vi "Rinocloud_browser.vi"() -> ()   [LabVIEW 2013, in "Rinocloud Library.lvlib"]
uses:
  Rinocloud Library.lvlib
  Rinocloud API endpoint VIs/API_endpoint_subVIs/State_Control.ctl
  Rinocloud_global_variable.vi
panel:
  in  "page indicator":string
  in  "Next page":bool
  in  "Previous page":bool
  out "Last action:":string
  in  "Active item:":string="<folder> home (id=)"
  in  "delete":bool
  in  "refresh list":bool
  in  "Tab Control":T1(tab)=enum."Inspect"
  in  "Cluster 2":T2={"Attribute"="", "Value"="", "Data type"=5} {"Data type" items=["Numeric", "String", "1D array of strings", "1D array of doubles", "Data JSON string", "<null>"]}
  in  "Cluster 1":T2={"Attribute"="", "Value"="", "Data type"=5} {"Data type" items=["Numeric", "String", "1D array of strings", "1D array of doubles", "Data JSON string", "<null>"]}
  in  "name":string
  in  "tags":string
  in  "notes":string
  in  "new folder":bool
  in  "upload file":bool
  in  "Store data locally":bool
  in  "Store metadata locally":bool
  in  "Name:":string
  in  "Tags:":string
  in  "Notes:":string
  in  "get metadata":bool
  in  "metadata tree":string(tree) caption="Metadata"
  in  "update metadata":bool
  in  "Move":bool
  in  "Destination:":string
  in  "Source:":string
  in  "set source":bool
  in  "set destination":bool
  out "body":string
  out "headers":string
  in  "error message":string caption="Error:"
  in  "ancestor tree":string(tree)="home" caption="Active path"
  in  "stop":bool
  in  "active child tree":string(tree) caption="File & folder list of the active folder"
  # "Double-click an item to activate"
  # "Custom metadata:"
  # "(tag1,tag2,tag3,...)"
  # "Click the fields to edit"
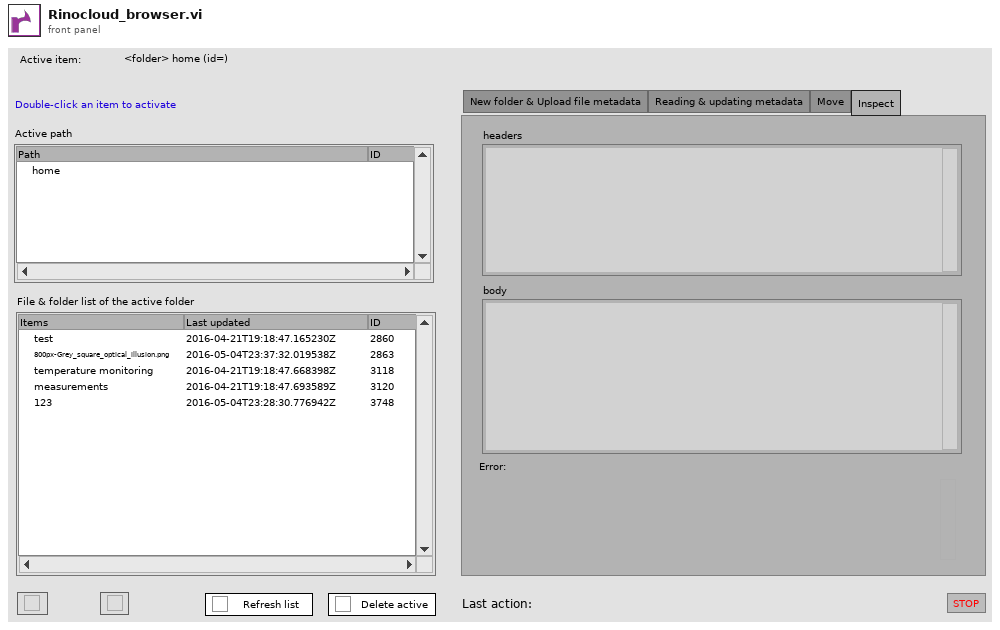
[diagram p1: front panel]
types:
  T1 = enum32{"New folder & Upload file metadata", "Reading & updating metadata", "Move", "Inspect"}
  T2 = cluster{"Attribute":string, "Value":string, "Data type":u16}
  T3 = cluster{"Active items":cluster{"Active file ID":string, "Active dir ID":string, "Active object ID":string, "Recent ID":string, "Active item:":string, "Source item":string, "Destination item":string, "Source ID":string, "Destination ID":string}, "Trees":cluster{"Ancestors":refnum<vi>, "Children":refnum<vi>, "Metadata":refnum<vi>}, "New metadata":cluster{"Name":string, "Tags":string, "Notes":string, "Custom metadata":cluster{"Attribute":string, "Value":string, "Data type":u16}[]}, "Communication":cluster{"HTTP headers":string, "HTTP body":string, "Project name":string, "User":string, "HTTP ch body":string}, "Controls":cluster{"Move refnum":refnum<vi>}, "Status messages":cluster{"error ":errorcluster, "status":string}, "Update metadata":cluster{"Name":string, "Tags":string, "Notes":string}, "Pagination":cluster{"total":dbl, "limit":dbl, "offset":dbl, "count":dbl, " next page refnum":refnum<vi>, "previous page refnum":refnum<vi>, "page indicator":string}}
  T4 = typedef "State_Control.ctl" = enum16{"Boot", "Initialize", "Wait for event", "Refresh", "Pagination", "Metadata to tree", "Stop"}
  T5 = cluster{"HTTP headers":string, "HTTP body":string, "Project name":string, "User":string, "HTTP ch body":string}
  T6 = cluster{"Active file ID":string, "Active dir ID":string, "Active object ID":string, "Recent ID":string, "Active item:":string, "Source item":string, "Destination item":string, "Source ID":string, "Destination ID":string}
  T7 = enum8{"Enabled", "Disabled", "Disabled and Grayed Out"}
  T8 = cluster{"Name":string, "Tags":string, "Notes":string, "Custom metadata":cluster{"Attribute":string, "Value":string, "Data type":u16}[]}
  T9 = enum16{"Boot", "Initialize", "Wait for event", "Refresh", "Pagination", "Metadata to tree", "Stop"}
  T10 = cluster{"Store locally":bool, "ancestor array":cluster{"id":string, "name":string, "created_on":string, "updated_on":string, "tags":string, "notes":string, "record type":string, "metadata (JSON)":string}[], "Store metadata":bool}
  T11 = cluster{"Attribute":string, "Value":string, "Data type":enum16{"Numeric", "String", "1D array of strings", "1D array of doubles", "Data JSON string", "<null>"}}[]
  T12 = cluster{"limit":dbl, "total":dbl, "offset":dbl, "count":dbl}
  T13 = cluster{"headers":string, "body":string, "ID":string, "Saved":bool}
  T14 = cluster{"Attribute":string, "Value":string, "Data type":u16}[]
  T15 = cluster{"id":string, "name":string, "created_on":string, "updated_on":string, "tags":string, "notes":string, "record type":string, "metadata (JSON)":string}[]
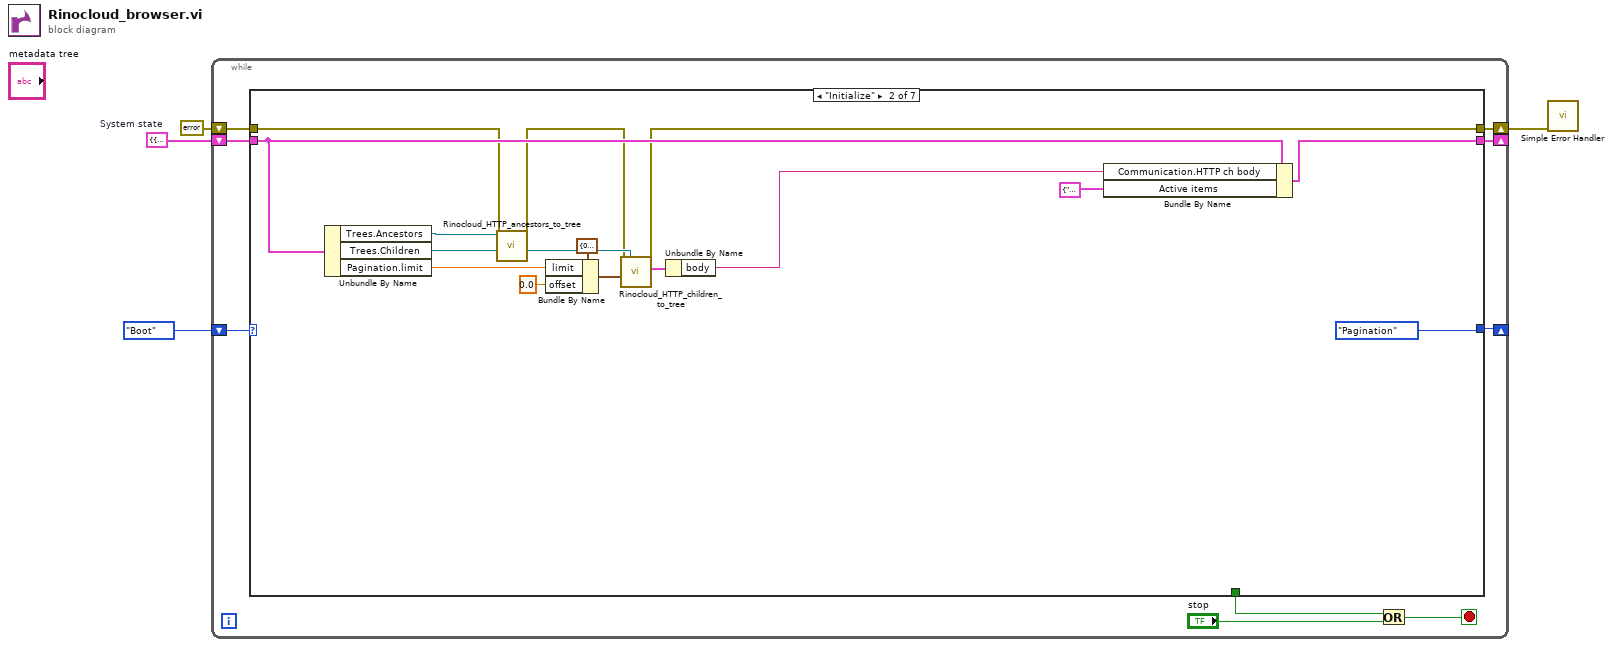
[diagram p0: block diagram]
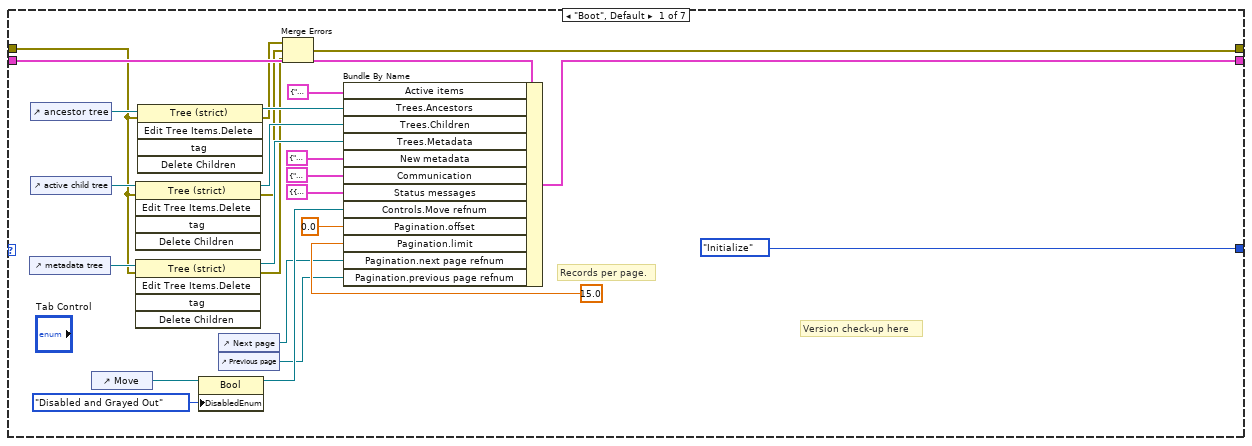
[diagram p2: hidden frame]
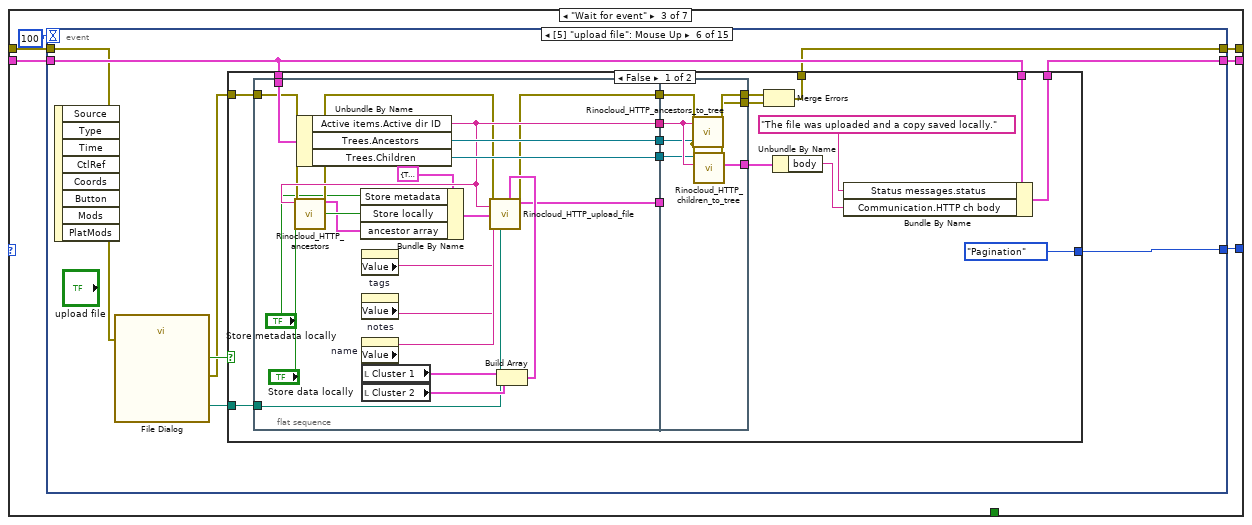
[diagram p3: hidden frame]
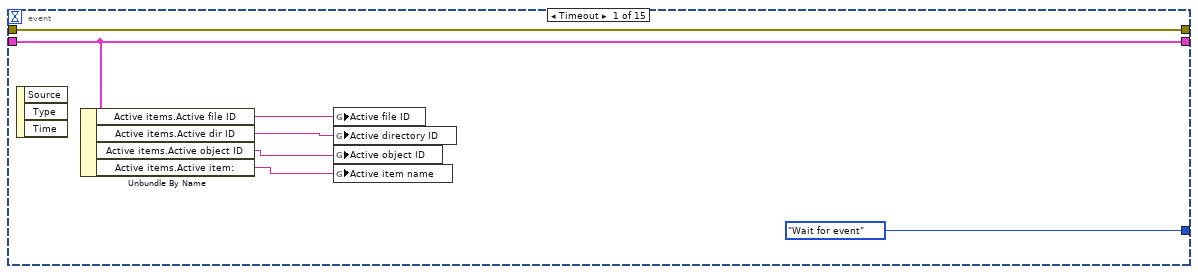
[diagram p4: hidden frame]
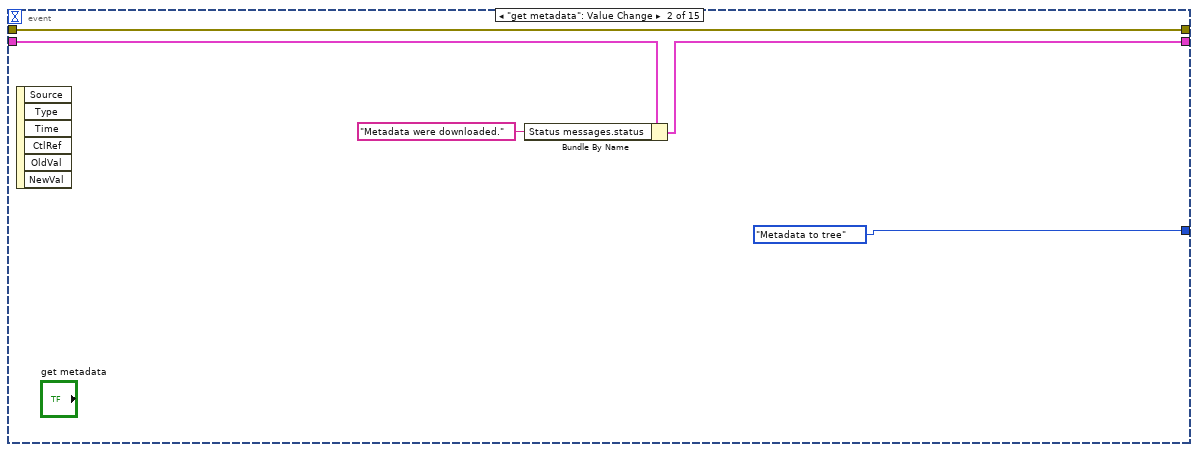
[diagram p5: hidden frame]
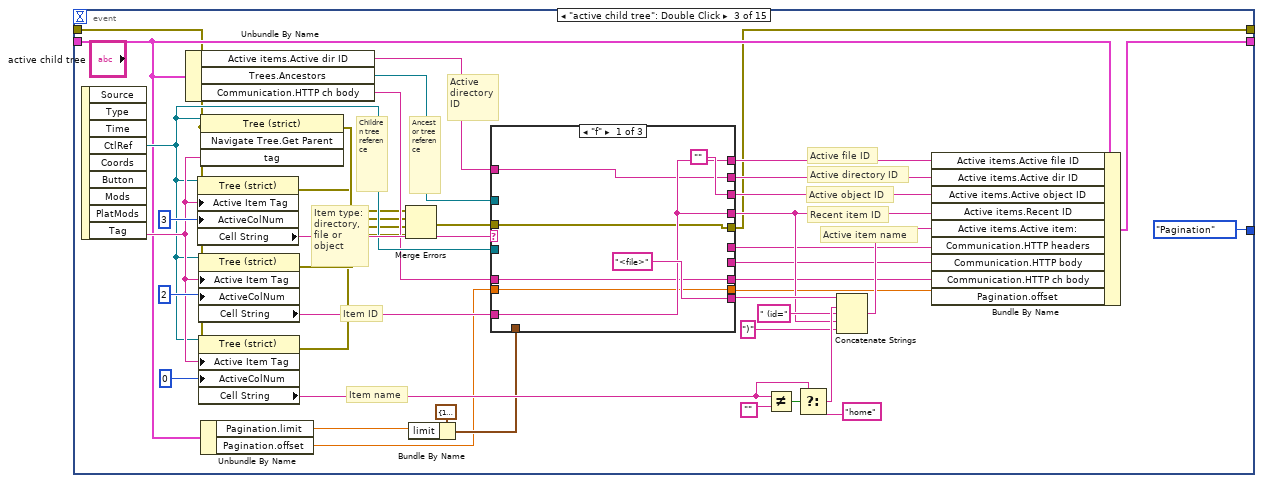
[diagram p6: hidden frame]
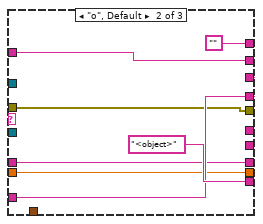
[diagram p7: hidden frame]
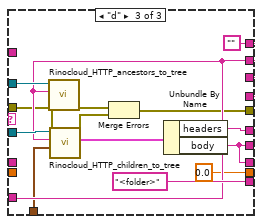
[diagram p8: hidden frame]
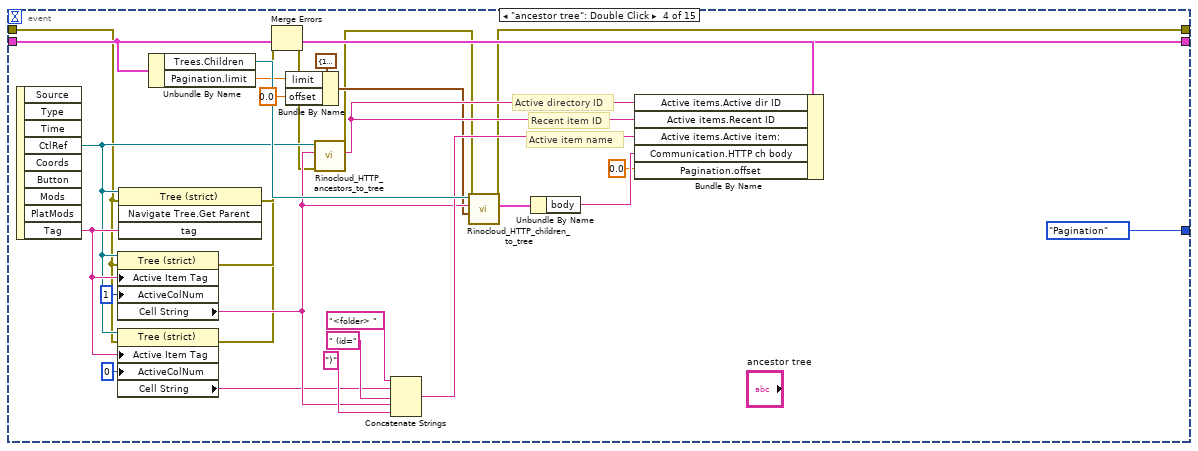
[diagram p9: hidden frame]
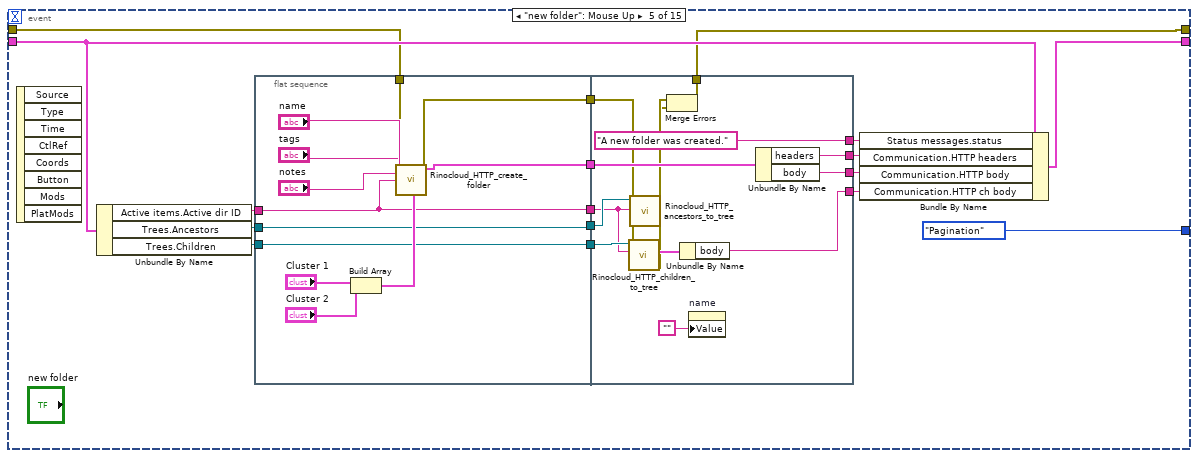
[diagram p10: hidden frame]
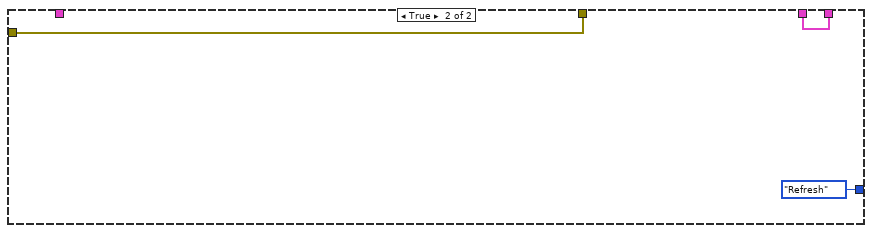
[diagram p11: hidden frame]
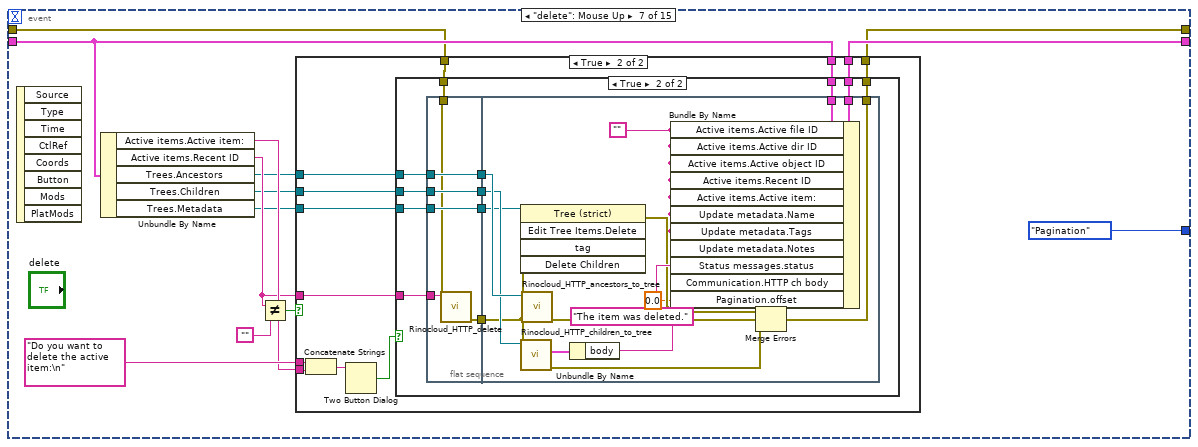
[diagram p12: hidden frame]
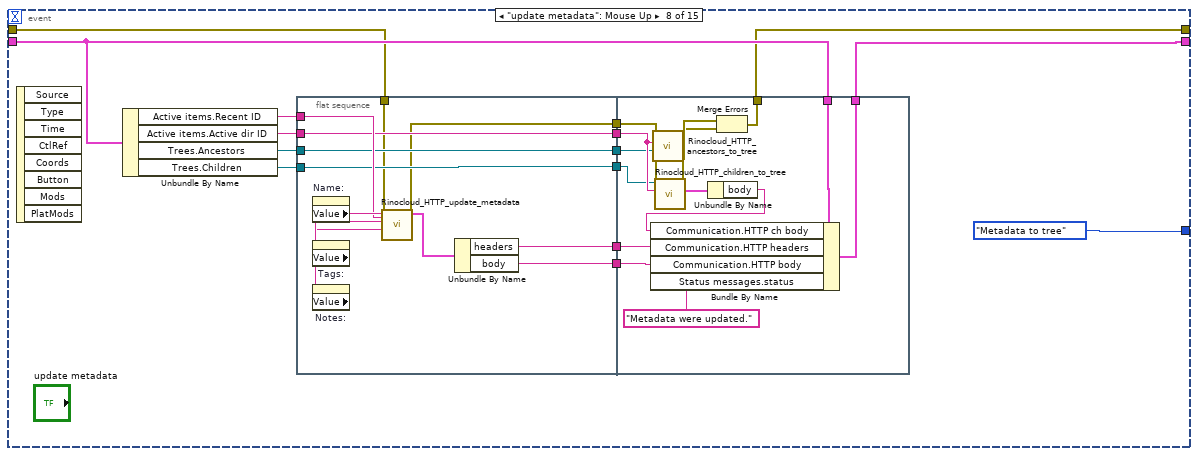
[diagram p15: hidden frame]
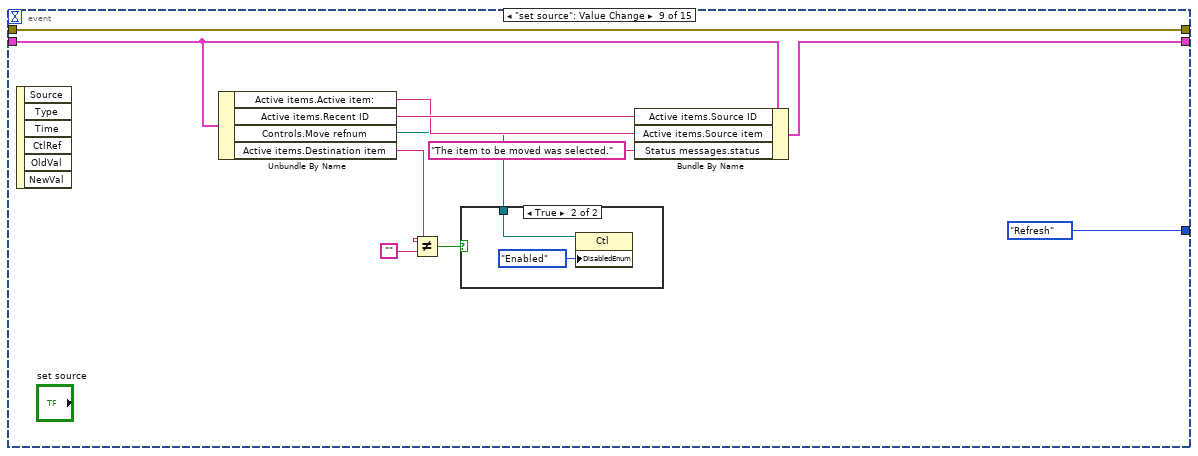
[diagram p16: hidden frame]
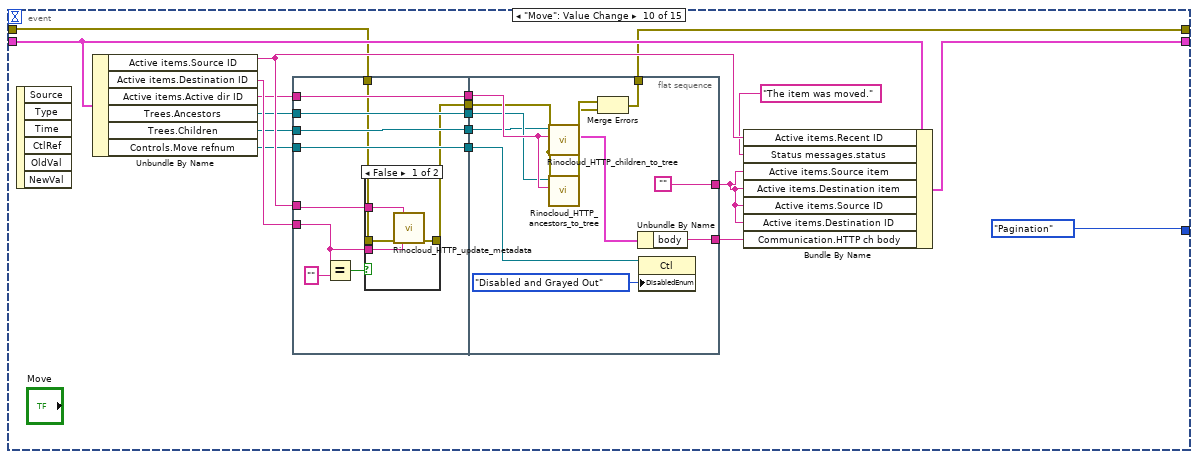
[diagram p18: hidden frame]
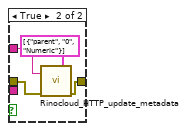
[diagram p19: hidden frame]
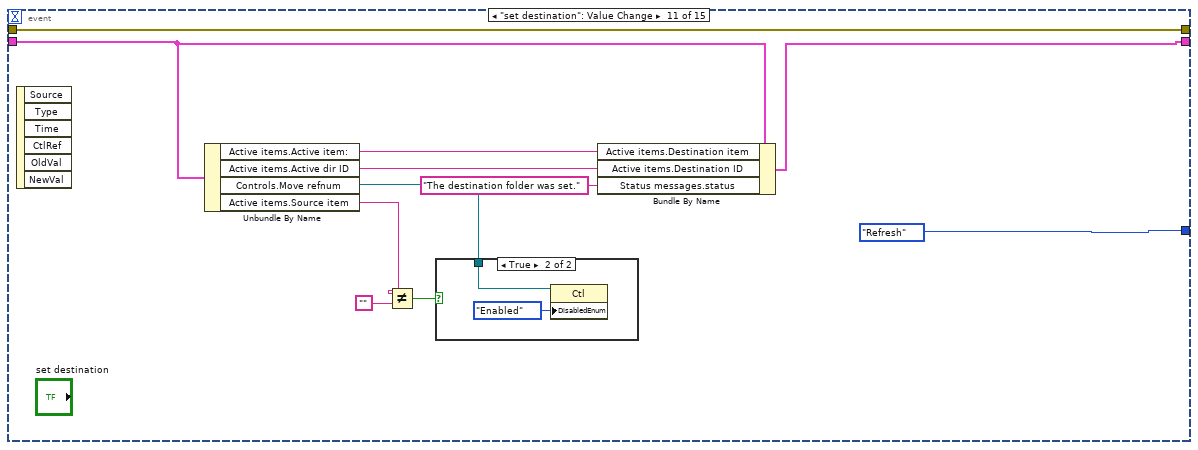
[diagram p20: hidden frame]
diagram:
  w4 = T3 {"Active items"={"Active file ID"="", "Active dir ID"="", "Active object ID"="", "Recent ID"="", "Active item:"="<folder> home (id=)", "Source item"="", "Destination item"="", "Source ID"="", "Destination ID"=""}, "Trees"={"Ancestors"=refnum, "Children"=refnum, "Metadata"=refnum}, "New metadata"={"Name"="", "Tags"="", "Notes"="", "Custom metadata"=[]}, "Communication"={"HTTP headers"="", "HTTP body"="", "Project name"="", "User"="", "HTTP ch body"=""}, "Controls"={"Move refnum"=refnum}, "Status messages"={"error "={"status"=FALSE, "code"=0, "source"=""}, "status"=""}, "Update metadata"={"Name"="", "Tags"="", "Notes"=""}, "Pagination"={"total"=0.0, "limit"=0.0, "offset"=0.0, "count"=0.0, " next page refnum"=refnum, "previous page refnum"=refnum, "page indicator"=""}}  # System state
  n1 = while {
    shift-right: [w7] -> _
    shift-left: State_Control."Boot" -> [w13]
    shift-right: [w8] -> _
    shift-left: w4 -> [w9]
    shift-right: [w5] -> w1
    shift-left: errorcluster {"status"=FALSE, "code"=0, "source"=""} ("errors") -> [w6]
    stop <- w12 stop-if-true
    n2 = case shown="\"Initialize\"" w13 {
      tunnel: [State_Control."Initialize" T9."Pagination" w58 T9."Wait for event" T9."Metadata to tree" T9."Refresh" T9."Metadata to tree"] -> w7
      tunnel: [_ _ _ _ TRUE _ _] -> w10
      tunnel: w9 -> [w38 w50 w57 w493 w499 w509 w538]
      tunnel: [w30 w49 w56 w493 w499 w508 w537] -> w8
      tunnel: w6 -> [w21 w43 w55 w481 w497 w502 w536]
      tunnel: [w17 w41 w54 _ w497 w501 w535] -> w5
      frame "Boot", Default {
        # "Records per page."
        # "Version check-up here"
        n3 = control-ref of="metadata tree"() -> (w33:refnum<vi>)
        n4 = control-ref of="ancestor tree"() -> (w37:refnum<vi>)
        n5 = control-ref of="active child tree"() -> (w35:refnum<vi>)
        n6 = control-ref of="Move"() -> (w29:refnum<vi>)
        n7 = invoke class="Tree (strict)" method="Edit Tree Items.Delete"(reference=w35, error in=w21) -> (reference out=w34:refnum<vi>, error out=w19:errorcluster)  [unwired: 3 in, 3 out]
        n8 = invoke class="Tree (strict)" method="Edit Tree Items.Delete"(reference=w33, error in=w21) -> (reference out=w25:refnum<vi>, error out=w18:errorcluster)  [unwired: 3 in, 3 out]
        n9 = invoke class="Tree (strict)" method="Edit Tree Items.Delete"(reference=w37, error in=w21) -> (reference out=w36:refnum<vi>, error out=w20:errorcluster)  [unwired: 3 in, 3 out]
        n10 = property class="Bool"(reference=w29, "DisabledEnum"=T7."Disabled and Grayed Out" ("Disabled")) -> (reference out=w27:refnum<vi>)  [unwired: 1 in, 1 out]
        n11 = control-ref of="Next page"() -> (w15:refnum<vi>)
        n12 = control-ref of="Previous page"() -> (w14:refnum<vi>)
        n13 = Merge Errors(w20, w19, w18) -> (w17:errorcluster)
        n14 = Bundle By Name(cluster=w38, "Active items"=T6 {"Active file ID"="", "Active dir ID"="", "Active object ID"="", "Recent ID"="", "Active item:"="<folder> home (id=)", "Source item"="", "Destination item"="", "Source ID"="", "Destination ID"=""}, "Trees.Ancestors"=w36, "Trees.Children"=w34, "Trees.Metadata"=w25, "New metadata"=T8 {"Name"="", "Tags"="", "Notes"="", "Custom metadata"=[]} ("Metadata"), "Communication"=T5 {"HTTP headers"="", "HTTP body"="", "Project name"="", "User"="", "HTTP ch body"=""}, "Status messages"=cluster{"error ":errorcluster, "status":string} {"error "={"status"=FALSE, "code"=0, "source"=""}, "status"=""}, "Controls.Move refnum"=w27, "Pagination.offset"=0.0, "Pagination.limit"=15.0, "Pagination.next page refnum"=w15, "Pagination.previous page refnum"=w14) -> (w30:T3)
      }
      frame "Initialize" {
        n15 = Unbundle By Name(w50) -> ("Trees.Ancestors"=w51:refnum<vi>, "Trees.Children"=w52:refnum<vi>, "Pagination.limit"=w44:dbl)
        n16 = call "Rinocloud_HTTP_ancestors_to_tree.vi"("error in (no error)"=w43, "Tree Ref in"=w51) -> ("error out"=w42:errorcluster)  [unwired: 2 in, 3 out]
        n17 = Bundle By Name(cluster=cluster{"limit":dbl, "offset":dbl} {"limit"=0.0, "offset"=0.0} ("Pagination variables"), "limit"=w44, "offset"=0.0) -> (w45:cluster{"limit":dbl, "offset":dbl})
        n18 = call "Rinocloud_HTTP_children_to_tree.vi"("error in (no error)"=w42, "Pagination variables"=w45, "Tree Ref in"=w52) -> ("error out"=w41:errorcluster, "Status"=w53:T13)  [unwired: 6 in, 1 out]
        n19 = Unbundle By Name(w53) -> ("body"=w47:string)
        n20 = Bundle By Name(cluster=w50, "Communication.HTTP ch body"=w47, "Active items"=T6 {"Active file ID"="", "Active dir ID"="", "Active object ID"="", "Recent ID"="", "Active item:"="<folder> home (id=)", "Source item"="", "Destination item"="", "Source ID"="", "Destination ID"=""}) -> (w49:T3)
      }
      frame "Wait for event" {
        n21 = event shown="[5] \"upload file\": Mouse Up" {
          selector: _ -> [_ _ _ _ _ _ _ _ _ _ _ _ _ _ _]
          dyn-events: _ -> [_ _ _ _ _ _ _ _ _ _ _ _ _ _ _]
          timeout: 100 -> [_ _ _ _ _ _ _ _ _ _ _ _ _ _ _]
          tunnel: [T9."Wait for event" T9."Metadata to tree" T9."Pagination" T9."Pagination" T9."Pagination" w213 T9."Pagination" T9."Metadata to tree" T9."Refresh" T9."Pagination" T9."Refresh" T9."Initialize" T9."Stop" T9."Pagination" T9."Pagination"] -> w58
          tunnel: w57 -> [w62 w70 w88 w165 w180 w218 w272 w337 w381 w401 w438 w450 _ w466 w479]
          tunnel: [w62 w69 w99 w163 w179 w217 w271 w334 w374 w392 w435 w449 _ w464 w478] -> w56
          tunnel: w55 -> [w60 w67 w80 w149 w172 w216 w269 w332 w371 w386 w433 w447 _ w454 w468]
          tunnel: [w60 w67 w74 w143 w170 w214 w268 w330 w371 w384 w433 w447 _ w453 w467] -> w54
          event Timeout {
            n22 = event-data() -> ()  [unwired: 1 in, 3 out]
            n23 = Unbundle By Name(w62) -> ("Active items.Active file ID"=w66:string, "Active items.Active dir ID"=w65:string, "Active items.Active object ID"=w64:string, "Active items.Active item:"=w63:string)
            n24 = global write "Rinocloud_global_variable.vi" "Active file ID"(w66) -> ()
            n25 = global write "Rinocloud_global_variable.vi" "Active directory ID"(w65) -> ()
            n26 = global write "Rinocloud_global_variable.vi" "Active object ID"(w64) -> ()
            n27 = global write "Rinocloud_global_variable.vi" "Active item name"(w63) -> ()
          }
          event "get metadata": Value Change {
            n28 = event-data() -> ()  [unwired: 1 in, 6 out]
            n29 = Bundle By Name(cluster=w70, "Status messages.status"="Metadata were downloaded.") -> (w69:T3)
          }
          event "active child tree": Double Click {
            # "Active \ndirectory\nID"
            # "Ancestor tree \nreference"
            # "Children tree \nreference"
            # "Item name"
            # "Item type:\ndirectory,\nfile or\nobject"
            # "Item ID"
            # "Active item name"
            # "Recent item ID"
            # "Active object ID"
            # "Active directory ID"
            # "Active file ID"
            n30 = event-data() -> ("CtlRef"=w90:refnum<vi>, "Tag"=w95:string)  [unwired: 1 in, 7 out]
            n31 = Unbundle By Name(w88) -> ("Active items.Active dir ID"=w100:string, "Trees.Ancestors"=w101:refnum<vi>, "Communication.HTTP ch body"=w84:string)
            n32 = property on="Property Node" class="Tree (strict)"(reference=w90, error in=w80, "Active Item Tag"=w95, "ActiveColNum"=3 ("Active Cell:Active Column Number")) -> (error out=w78:errorcluster, "Cell String"=w94:string)  [unwired: 1 out]
            n33 = property on="Property Node" class="Tree (strict)"(reference=w90, error in=w80, "Active Item Tag"=w95, "ActiveColNum"=2 ("Active Cell:Active Column Number")) -> (error out=w77:errorcluster, "Cell String"=w93:string)  [unwired: 1 out]
            n34 = property on="Property Node" class="Tree (strict)"(reference=w90, error in=w80, "Active Item Tag"=w95, "ActiveColNum"=0 ("Active Cell:Active Column Number")) -> (error out=w76:errorcluster, "Cell String"=w92:string)  [unwired: 1 out]
            n35 = invoke on="Invoke Node" class="Tree (strict)" method="Navigate Tree.Get Parent"(reference=w90, error in=w80, "tag"=w95) -> (error out=w79:errorcluster)  [unwired: 1 in, 3 out]
            n36 = Unbundle By Name(w88) -> ("Pagination.limit"=w86:dbl, "Pagination.offset"=w72:dbl)
            n37 = Merge Errors(w79, w78, w77, w76) -> (w75:errorcluster)
            n38 = Bundle By Name(cluster=cluster{"limit":dbl, "offset":dbl} {"limit"=15.0, "offset"=0.0} ("Pagination variables"), "limit"=w86) -> (w85:cluster{"limit":dbl, "offset":dbl})
            n39 = case shown="\"f\"" w94 {
              tunnel: w93 -> [w117 w125 w136]
              tunnel: ["<file>" ("f") "<object>" ("f") "<folder>" ("f")] -> w109
              tunnel: [w117 w125 w136] -> w103
              tunnel: ["" w125 w139] -> w104
              tunnel: [w117 "" w139] -> w91
              tunnel: [w116 w123 w136] -> w102
              tunnel: w101 -> [_ _ w138]
              tunnel: w90 -> [_ _ w137]
              tunnel: w100 -> [w116 w123 _]
              tunnel: w85 -> [_ _ w135]
              tunnel: w84 -> [w115 w122 _]
              tunnel: [w115 w122 w132] -> w83
              tunnel: [_ _ w132] -> w82
              tunnel: [_ _ w133] -> w81
              tunnel: w75 -> [w114 w121 w131]
              tunnel: [w114 w121 w128] -> w74
              tunnel: [w113 w120 0.0 ("Pagination.offset")] -> w73
              tunnel: w72 -> [w113 w120 _]
              frame "f" {
              }
              frame "o", Default {
              }
              frame "d" {
                w139 = ""
                n40 = call "Rinocloud_HTTP_ancestors_to_tree.vi"("error in (no error)"=w131, "id"=w136, "Tree Ref in"=w138) -> ("error out"=w130:errorcluster)  [unwired: 1 in, 3 out]
                n41 = call "Rinocloud_HTTP_children_to_tree.vi"("error in (no error)"=w131, "Pagination variables"=w135, "id"=w136, "Tree Ref in"=w137) -> ("error out"=w129:errorcluster, "Status"=w134:T13)  [unwired: 5 in, 1 out]
                n42 = Merge Errors(w130, w129) -> (w128:errorcluster)
                n43 = Unbundle By Name(w134) -> ("headers"=w133:string, "body"=w132:string)
              }
            }
            n44 = Not Equal?(x=w92, y="") -> (x != y?=w111:bool)
            n45 = Select(t=w92, s=w111, f="home") -> (s? t:f=w108:string)
            n46 = Concatenate Strings(w109, w108, " (id=" ("string"), w103, ")" ("string")) -> (w105:string)
            n47 = Bundle By Name(cluster=w88, "Active items.Active file ID"=w91, "Active items.Active dir ID"=w102, "Active items.Active object ID"=w104, "Active items.Recent ID"=w103, "Active items.Active item:"=w105, "Communication.HTTP headers"=w81, "Communication.HTTP body"=w82, "Communication.HTTP ch body"=w83, "Pagination.offset"=w73) -> (w99:T3)
          }
          event "ancestor tree": Double Click {
            # "Active item name"
            # "Recent item ID"
            # "Active directory ID"
            n48 = event-data() -> ("CtlRef"=w156:refnum<vi>, "Tag"=w159:string)  [unwired: 1 in, 7 out]
            n49 = property on="Property Node" class="Tree (strict)"(reference=w156, error in=w149, "Active Item Tag"=w159, "ActiveColNum"=1 ("Active Cell:Active Column Number")) -> (error out=w147:errorcluster, "Cell String"=w158:string)  [unwired: 1 out]
            n50 = property on="Property Node" class="Tree (strict)"(reference=w156, error in=w149, "Active Item Tag"=w159, "ActiveColNum"=0 ("Active Cell:Active Column Number")) -> (error out=w146:errorcluster, "Cell String"=w157:string)  [unwired: 1 out]
            n51 = invoke on="Invoke Node" class="Tree (strict)" method="Navigate Tree.Get Parent"(reference=w156, error in=w149, "tag"=w159) -> (error out=w148:errorcluster)  [unwired: 1 in, 3 out]
            n52 = Unbundle By Name(w165) -> ("Trees.Children"=w166:refnum<vi>, "Pagination.limit"=w152:dbl)
            n53 = Merge Errors(w148, w147, w146) -> (w145:errorcluster)
            n54 = Bundle By Name(cluster=cluster{"limit":dbl, "offset":dbl} {"limit"=15.0, "offset"=0.0} ("Pagination variables"), "limit"=w152, "offset"=0.0) -> (w153:cluster{"limit":dbl, "offset":dbl})
            n55 = call "Rinocloud_HTTP_ancestors_to_tree.vi"("error in (no error)"=w145, "id"=w158, "Tree Ref in"=w156) -> ("error out"=w144:errorcluster, "last ID"=w164:string)  [unwired: 1 in, 2 out]
            n56 = Concatenate Strings("<folder> " ("string"), w157, " (id=" ("string"), w158, ")" ("string")) -> (w162:string)
            n57 = call "Rinocloud_HTTP_children_to_tree.vi"("error in (no error)"=w144, "Pagination variables"=w153, "id"=w158, "Tree Ref in"=w166) -> ("error out"=w143:errorcluster, "Status"=w151:T13)  [unwired: 5 in, 1 out]
            n58 = Unbundle By Name(w151) -> ("body"=w150:string)
            n59 = Bundle By Name(cluster=w165, "Active items.Active dir ID"=w164, "Active items.Recent ID"=w164, "Active items.Active item:"=w162, "Communication.HTTP ch body"=w150, "Pagination.offset"=0.0) -> (w163:T3)
          }
          event "new folder": Mouse Up {
            n60 = event-data() -> ()  [unwired: 1 in, 8 out]
            n61 = Unbundle By Name(w180) -> ("Active items.Active dir ID"=w186:string, "Trees.Ancestors"=w185:refnum<vi>, "Trees.Children"=w184:refnum<vi>)
            n62 = flat-sequence {
              tunnel: w186 -> [w197]
              tunnel: w185 -> [w196]
              tunnel: w184 -> [w195]
              tunnel: [w197] -> w183
              tunnel: [w196] -> w182
              tunnel: [w195] -> w181
              tunnel: [w194] -> w178
              tunnel: w172 -> [w188]
              tunnel: [w187] -> w171
              tunnel: w183 -> [w209]
              tunnel: w182 -> [w211]
              tunnel: w181 -> [w210]
              tunnel: w178 -> [w208]
              tunnel: [w207] -> w177
              tunnel: [w206] -> w176
              tunnel: ["A new folder was created." ("Status messages.status")] -> w175
              tunnel: [w203] -> w173
              tunnel: w171 -> [w202]
              tunnel: [w199] -> w170
              frame #0 {
                n63 = Build Array("Cluster 1", "Cluster 2") -> (w198:T14)
                n64 = call "Rinocloud_HTTP_create_folder.vi"("Extra metadata array"=w198, "Parent ID"=w197, "error in (no error)"=w188, "Notes"="notes", "Tags"="tags", "Name"="name") -> ("error out"=w187:errorcluster, "Status"=w194:T13)  [unwired: 2 in]
              }
              frame #1 {
                n65 = call "Rinocloud_HTTP_children_to_tree.vi"("error in (no error)"=w202, "id"=w209, "Tree Ref in"=w210) -> ("error out"=w200:errorcluster, "Status"=w204:T13)  [unwired: 6 in, 1 out]
                n66 = call "Rinocloud_HTTP_ancestors_to_tree.vi"("error in (no error)"=w202, "id"=w209, "Tree Ref in"=w211) -> ("error out"=w201:errorcluster)  [unwired: 1 in, 3 out]
                n67 = Merge Errors(w201, w200) -> (w199:errorcluster)
                n68 = Unbundle By Name(w204) -> ("body"=w203:string)
                n69 = property on="name" class="Str"("Value"="") -> ()  [unwired: 2 in, 2 out]
                n70 = Unbundle By Name(w208) -> ("headers"=w207:string, "body"=w206:string)
              }
            }
            n71 = Bundle By Name(cluster=w180, "Status messages.status"=w175, "Communication.HTTP headers"=w177, "Communication.HTTP body"=w176, "Communication.HTTP ch body"=w173) -> (w179:T3)
          }
          event "upload file": Mouse Up {
            n72 = event-data() -> ()  [unwired: 1 in, 8 out]
            n73 = call "File Dialog"("error in"=w216) -> ("selected path"=w219:path, "cancelled"=w220:bool, "error out"=w215:errorcluster)  [unwired: 11 in, 1 out]
            n74 = case shown="False" w220 {
              tunnel: w219 -> [w237 _]
              tunnel: w218 -> [w236 _]
              tunnel: w218 -> [w231 w267]
              tunnel: [w229 w267] -> w217
              tunnel: w215 -> [w226 w266]
              tunnel: [w222 w266] -> w214
              tunnel: [T9."Pagination" T9."Refresh"] -> w213
              frame False {
                n75 = flat-sequence {
                  tunnel: w237 -> [w255]
                  tunnel: w236 -> [w248]
                  tunnel: [w247] -> w235
                  tunnel: [w246] -> w234
                  tunnel: [w245] -> w233
                  tunnel: [w244] -> w232
                  tunnel: w226 -> [w241]
                  tunnel: [w239] -> w225
                  tunnel: w235 -> [w262]
                  tunnel: w234 -> [w263]
                  tunnel: w233 -> [_]
                  tunnel: w232 -> [w264]
                  tunnel: [w261] -> w228
                  tunnel: w225 -> [w260]
                  tunnel: [w259] -> w224
                  tunnel: [w258] -> w223
                  frame #0 {
                    n76 = Unbundle By Name(w248) -> ("Active items.Active dir ID"=w244:string, "Trees.Ancestors"=w247:refnum<vi>, "Trees.Children"=w246:refnum<vi>)
                    n77 = call "Rinocloud_HTTP_ancestors.vi"("error in (no error)"=w241, "id"=w244) -> ("error out"=w240:errorcluster, "metadata array"=w249:T15)  [unwired: 2 in, 2 out]
                    n78 = Bundle By Name(cluster=T10 {"Store locally"=TRUE, "ancestor array"=[], "Store metadata"=TRUE} ("local storage"), "Store metadata"="Store metadata locally", "Store locally"="Store data locally", "ancestor array"=w249) -> (w242:T10)
                    n79 = property on="tags" class="Str"() -> ("Value"=w253:string)  [unwired: 2 in, 2 out]
                    n80 = property on="notes" class="Str"() -> ("Value"=w252:string)  [unwired: 2 in, 2 out]
                    n81 = property on="name" class="Str"() -> ("Value"=w254:string)  [unwired: 2 in, 2 out]
                    n82 = local read "Cluster 1"() -> (w257:T2)
                    n83 = local read "Cluster 2"() -> (w256:T2)
                    n84 = Build Array(w257, w256) -> (w251:T14)
                    n85 = call "Rinocloud_HTTP_upload_file.vi"("local storage"=w242, "Extra metadata array"=w251, "Path in"=w255, "Parent ID"=w244, "error in (no error)"=w240, "Notes"=w252, "Tags"=w253, "Name"=w254) -> ("error out"=w239:errorcluster, "Status"=w245:T13)  [unwired: 1 in, 1 out]
                  }
                  frame #1 {
                    n86 = call "Rinocloud_HTTP_ancestors_to_tree.vi"("error in (no error)"=w260, "id"=w264, "Tree Ref in"=w262) -> ("error out"=w259:errorcluster)  [unwired: 1 in, 3 out]
                    n87 = call "Rinocloud_HTTP_children_to_tree.vi"("error in (no error)"=w260, "id"=w264, "Tree Ref in"=w263) -> ("error out"=w258:errorcluster, "Status"=w261:T13)  [unwired: 6 in, 1 out]
                  }
                }
                n88 = Merge Errors(w224, w223) -> (w222:errorcluster)
                n89 = Unbundle By Name(w228) -> ("body"=w227:string)
                n90 = Bundle By Name(cluster=w231, "Status messages.status"="The file was uploaded and a copy saved locally.", "Communication.HTTP ch body"=w227) -> (w229:T3)
              }
              frame True {
              }
            }
          }
          event "delete": Mouse Up {
            n91 = event-data() -> ()  [unwired: 1 in, 8 out]
            n92 = Unbundle By Name(w272) -> ("Active items.Active item:"=w277:string, "Active items.Recent ID"=w276:string, "Trees.Ancestors"=w275:refnum<vi>, "Trees.Children"=w274:refnum<vi>, "Trees.Metadata"=w273:refnum<vi>)
            n93 = Not Equal?(x=w276, y="") -> (x != y?=w280:bool)
            n94 = case shown="True" w280 {
              tunnel: w276 -> [_ w292]
              tunnel: "Do you want to delete the active item:\n" ("message") -> [_ w291]
              tunnel: w277 -> [_ w290]
              tunnel: w275 -> [_ w289]
              tunnel: w274 -> [_ w288]
              tunnel: w273 -> [_ w287]
              tunnel: w272 -> [w282 w286]
              tunnel: [w282 w285] -> w271
              tunnel: w269 -> [w281 w284]
              tunnel: [w281 w283] -> w268
              frame False {
              }
              frame True {
                n95 = Concatenate Strings(w291, w290) -> (w294:string)
                n96 = Two Button Dialog(message=w294) -> (T button?=w293:bool)  [unwired: 2 in]
                n97 = case shown="True" w293 {
                  tunnel: w292 -> [_ w308]
                  tunnel: w289 -> [_ w306]
                  tunnel: w288 -> [_ w304]
                  tunnel: w287 -> [_ w302]
                  tunnel: w286 -> [w296 w301]
                  tunnel: [w296 w300] -> w285
                  tunnel: w284 -> [w295 w299]
                  tunnel: [w295 w297] -> w283
                  frame False {
                  }
                  frame True {
                    n98 = flat-sequence {
                      tunnel: w308 -> [w314]
                      tunnel: [w313] -> w307
                      tunnel: w306 -> [w313]
                      tunnel: [w312] -> w305
                      tunnel: w304 -> [w312]
                      tunnel: [w311] -> w303
                      tunnel: w302 -> [w311]
                      tunnel: w299 -> [w310]
                      tunnel: [w309] -> w298
                      tunnel: w307 -> [w329]
                      tunnel: w305 -> [w328]
                      tunnel: w303 -> [w327]
                      tunnel: w301 -> [w326]
                      tunnel: [w323] -> w300
                      tunnel: w298 -> [w320]
                      tunnel: [w316] -> w297
                      frame #0 {
                        n99 = call "Rinocloud_HTTP_delete.vi"("error in (no error)"=w310, "ID"=w314) -> ("error out"=w309:errorcluster)  [unwired: 5 in, 1 out]
                      }
                      frame #1 {
                        w325 = ""
                        n100 = invoke class="Tree (strict)" method="Edit Tree Items.Delete"(reference=w327, error in=w320) -> (error out=w319:errorcluster)  [unwired: 3 in, 4 out]
                        n101 = call "Rinocloud_HTTP_children_to_tree.vi"("error in (no error)"=w320, "Tree Ref in"=w328) -> ("error out"=w317:errorcluster, "Status"=w322:T13)  [unwired: 7 in, 1 out]
                        n102 = call "Rinocloud_HTTP_ancestors_to_tree.vi"("error in (no error)"=w320, "Tree Ref in"=w329) -> ("error out"=w318:errorcluster)  [unwired: 2 in, 3 out]
                        n103 = Unbundle By Name(w322) -> ("body"=w321:string)
                        n104 = Bundle By Name(cluster=w326, "Active items.Active file ID"=w325, "Active items.Active dir ID"=w325, "Active items.Active object ID"=w325, "Active items.Recent ID"=w325, "Active items.Active item:"=w325, "Update metadata.Name"=w325, "Update metadata.Tags"=w325, "Update metadata.Notes"=w325, "Status messages.status"="The item was deleted.", "Communication.HTTP ch body"=w321, "Pagination.offset"=0.0) -> (w323:T3)
                        n105 = Merge Errors(w319, w318, w317) -> (w316:errorcluster)
                      }
                    }
                  }
                }
              }
            }
          }
          event "update metadata": Mouse Up {
            n106 = event-data() -> ()  [unwired: 1 in, 8 out]
            n107 = Unbundle By Name(w337) -> ("Active items.Recent ID"=w344:string, "Active items.Active dir ID"=w342:string, "Trees.Ancestors"=w341:refnum<vi>, "Trees.Children"=w338:refnum<vi>)
            n108 = flat-sequence {
              tunnel: w344 -> [w353]
              tunnel: [w352] -> w343
              tunnel: w342 -> [w352]
              tunnel: w341 -> [w351]
              tunnel: [w351] -> w340
              tunnel: [w350] -> w339
              tunnel: w338 -> [w350]
              tunnel: [w348] -> w336
              tunnel: [w347] -> w335
              tunnel: w332 -> [w346]
              tunnel: [w345] -> w331
              tunnel: w343 -> [w370]
              tunnel: w340 -> [w368]
              tunnel: w339 -> [w369]
              tunnel: w337 -> [w367]
              tunnel: w336 -> [w365]
              tunnel: w335 -> [w364]
              tunnel: [w363] -> w334
              tunnel: w331 -> [w360]
              tunnel: [w357] -> w330
              frame #0 {
                n109 = property on="Name:" class="Str"() -> ("Value"=w354:string)  [unwired: 2 in, 2 out]
                n110 = property on="Tags:" class="Str"() -> ("Value"=w356:string)  [unwired: 2 in, 2 out]
                n111 = property on="Notes:" class="Str"() -> ("Value"=w355:string)  [unwired: 2 in, 2 out]
                n112 = call "Rinocloud_HTTP_update_metadata.vi"("self ID"=w353, "error in (no error)"=w346, "Notes"=w355, "Tags"=w356, "Name"=w354) -> ("error out"=w345:errorcluster, "Status"=w349:T13)  [unwired: 5 in]
                n113 = Unbundle By Name(w349) -> ("headers"=w348:string, "body"=w347:string)
              }
              frame #1 {
                n114 = call "Rinocloud_HTTP_ancestors_to_tree.vi"("error in (no error)"=w360, "id"=w370, "Tree Ref in"=w368) -> ("error out"=w359:errorcluster)  [unwired: 1 in, 3 out]
                n115 = call "Rinocloud_HTTP_children_to_tree.vi"("error in (no error)"=w360, "id"=w370, "Tree Ref in"=w369) -> ("error out"=w358:errorcluster, "Status"=w362:T13)  [unwired: 6 in, 1 out]
                n116 = Unbundle By Name(w362) -> ("body"=w361:string)
                n117 = Bundle By Name(cluster=w367, "Communication.HTTP ch body"=w361, "Communication.HTTP headers"=w365, "Communication.HTTP body"=w364, "Status messages.status"="Metadata were updated.") -> (w363:T3)
                n118 = Merge Errors(w359, w358) -> (w357:errorcluster)
              }
            }
          }
          event "set source": Value Change {
            n119 = event-data() -> ()  [unwired: 1 in, 6 out]
            n120 = Unbundle By Name(w381) -> ("Active items.Active item:"=w379:string, "Active items.Recent ID"=w380:string, "Controls.Move refnum"=w376:refnum<vi>, "Active items.Destination item"=w377:string)
            n121 = Not Equal?(x=w377, y="") -> (x != y?=w375:bool)
            n122 = case shown="True" w375 {
              tunnel: w376 -> [_ w382]
              frame False {
              }
              frame True {
                n123 = property class="Ctl"(reference=w382, "DisabledEnum"=T7."Enabled" ("Disabled")) -> ()  [unwired: 1 in, 2 out]
              }
            }
            n124 = Bundle By Name(cluster=w381, "Active items.Source ID"=w380, "Active items.Source item"=w379, "Status messages.status"="The item to be moved was selected.") -> (w374:T3)
          }
          event "Move": Value Change {
            n125 = event-data() -> ()  [unwired: 1 in, 6 out]
            n126 = Unbundle By Name(w401) -> ("Active items.Source ID"=w400:string, "Active items.Destination ID"=w402:string, "Active items.Active dir ID"=w398:string, "Trees.Ancestors"=w396:refnum<vi>, "Trees.Children"=w394:refnum<vi>, "Controls.Move refnum"=w390:refnum<vi>)
            n127 = flat-sequence {
              tunnel: w400 -> [w410]
              tunnel: w402 -> [w409]
              tunnel: [w408] -> w399
              tunnel: w398 -> [w408]
              tunnel: [w407] -> w397
              tunnel: w396 -> [w407]
              tunnel: [w406] -> w395
              tunnel: w394 -> [w406]
              tunnel: [w405] -> w391
              tunnel: w390 -> [w405]
              tunnel: w386 -> [w404]
              tunnel: [w403] -> w385
              tunnel: w399 -> [w432]
              tunnel: w397 -> [w431]
              tunnel: w395 -> [w430]
              tunnel: w391 -> [w429]
              tunnel: [""] -> w389
              tunnel: [w426] -> w387
              tunnel: w385 -> [w425]
              tunnel: [w422] -> w384
              frame #0 {
                n128 = Equal?(x=w409, y="") -> (x = y?=w411:bool)
                n129 = case shown="False" w411 {
                  tunnel: w410 -> [w416 w420]
                  tunnel: w409 -> [w415 _]
                  tunnel: w404 -> [w414 w418]
                  tunnel: [w413 w417] -> w403
                  frame False {
                    n130 = call "Rinocloud_HTTP_update_metadata.vi"("parent ID"=w415, "self ID"=w416, "error in (no error)"=w414) -> ("error out"=w413:errorcluster)  [unwired: 7 in, 1 out]
                  }
                  frame True {
                    n131 = call "Rinocloud_HTTP_update_metadata.vi"("Extra metadata array"=T11 [{"Attribute"="parent", "Value"="0", "Data type"=enum."Numeric"}], "self ID"=w420, "error in (no error)"=w418) -> ("error out"=w417:errorcluster)  [unwired: 7 in, 1 out]
                  }
                }
              }
              frame #1 {
                n132 = call "Rinocloud_HTTP_children_to_tree.vi"("error in (no error)"=w425, "id"=w432, "Tree Ref in"=w430) -> ("error out"=w424:errorcluster, "Status"=w421:T13)  [unwired: 6 in, 1 out]
                n133 = call "Rinocloud_HTTP_ancestors_to_tree.vi"("error in (no error)"=w425, "id"=w432, "Tree Ref in"=w431) -> ("error out"=w423:errorcluster)  [unwired: 1 in, 3 out]
                n134 = Merge Errors(w424, w423) -> (w422:errorcluster)
                n135 = Unbundle By Name(w421) -> ("body"=w426:string)
                n136 = property class="Ctl"(reference=w429, "DisabledEnum"=T7."Disabled and Grayed Out" ("Disabled")) -> ()  [unwired: 1 in, 2 out]
              }
            }
            n137 = Bundle By Name(cluster=w401, "Active items.Recent ID"=w400, "Status messages.status"="The item was moved.", "Active items.Source item"=w389, "Active items.Destination item"=w389, "Active items.Source ID"=w389, "Active items.Destination ID"=w389, "Communication.HTTP ch body"=w387) -> (w392:T3)
          }
          event "set destination": Value Change {
            n138 = event-data() -> ()  [unwired: 1 in, 6 out]
            n139 = Unbundle By Name(w438) -> ("Active items.Active item:"=w437:string, "Active items.Active dir ID"=w443:string, "Controls.Move refnum"=w440:refnum<vi>, "Active items.Source item"=w441:string)
            n140 = Not Equal?(x=w441, y="") -> (x != y?=w439:bool)
            n141 = case shown="True" w439 {
              tunnel: w440 -> [_ w444]
              frame False {
              }
              frame True {
                n142 = property class="Ctl"(reference=w444, "DisabledEnum"=T7."Enabled" ("Disabled")) -> ()  [unwired: 1 in, 2 out]
              }
            }
            n143 = Bundle By Name(cluster=w438, "Active items.Destination item"=w437, "Active items.Destination ID"=w443, "Status messages.status"="The destination folder was set.") -> (w435:T3)
          }
          event "refresh list": Mouse Up {
            n144 = event-data() -> ()  [unwired: 1 in, 8 out]
            n145 = Bundle By Name(cluster=w450, "Status messages.status"="The file list view was refreshed.", "Pagination.offset"=0.0) -> (w449:T3)
          }
          event "stop": Value Change {
            n146 = event-data() -> ()  [unwired: 1 in, 6 out]
          }
          event "Next page": Value Change {
            n147 = event-data() -> ()  [unwired: 1 in, 6 out]
            n148 = Unbundle By Name(w466) -> ("Pagination.limit"=w460:dbl, "Pagination.offset"=w465:dbl, "Active items.Active dir ID"=w462:string, "Trees.Children"=w455:refnum<vi>)
            n149 = Add(x=w460, y=w465) -> (x+y=w459:dbl)
            n150 = Bundle By Name(cluster=cluster{"limit":dbl, "offset":dbl} {"limit"=15.0, "offset"=0.0} ("Pagination variables"), "limit"=w460, "offset"=w459) -> (w458:cluster{"limit":dbl, "offset":dbl})
            n151 = call "Rinocloud_HTTP_children_to_tree.vi"("error in (no error)"=w454, "Pagination variables"=w458, "id"=w462, "Tree Ref in"=w455) -> ("error out"=w453:errorcluster, "Status"=w457:T13)  [unwired: 5 in, 1 out]
            n152 = Unbundle By Name(w457) -> ("body"=w456:string)
            n153 = Bundle By Name(cluster=w466, "Pagination.offset"=w459, "Communication.HTTP ch body"=w456) -> (w464:T3)
          }
          event "Previous page": Value Change {
            n154 = event-data() -> ()  [unwired: 1 in, 6 out]
            n155 = Unbundle By Name(w479) -> ("Pagination.offset"=w480:dbl, "Pagination.limit"=w473:dbl, "Active items.Active dir ID"=w474:string, "Trees.Children"=w469:refnum<vi>)
            n156 = Subtract(x=w480, y=w473) -> (x-y=w472:dbl)
            n157 = Bundle By Name(cluster=cluster{"limit":dbl, "offset":dbl} {"limit"=15.0, "offset"=0.0} ("Pagination variables"), "limit"=w473, "offset"=w472) -> (w475:cluster{"limit":dbl, "offset":dbl})
            n158 = call "Rinocloud_HTTP_children_to_tree.vi"("error in (no error)"=w468, "Pagination variables"=w475, "id"=w474, "Tree Ref in"=w469) -> ("error out"=w467:errorcluster, "Status"=w471:T13)  [unwired: 5 in, 1 out]
            n159 = Unbundle By Name(w471) -> ("body"=w470:string)
            n160 = Bundle By Name(cluster=w479, "Pagination.offset"=w472, "Communication.HTTP ch body"=w470) -> (w478:T3)
          }
        }
      }
      frame "Refresh" {
        n161 = Unbundle By Name(w493) -> ("Update metadata.Name"=w487:string, "Update metadata.Tags"=w486:string, "Update metadata.Notes"=w485:string, "Communication.HTTP headers"=→"headers":string, "Communication.HTTP body"=→"body":string, "Status messages.status"=→"Last action:":string, "Active items.Active item:"=w490:string, "Active items.Source item"=w489:string, "Active items.Destination item"=w488:string, "Pagination.page indicator"=w483:string)
        n162 = Unbundle By Name(w481) -> ("source"=w482:string)
        n163 = local write "error message"(w482) -> ()
        n164 = local write "Name:"(w487) -> ()
        n165 = local write "Tags:"(w486) -> ()
        n166 = local write "Notes:"(w485) -> ()
        n167 = local write "Active item:"(w490) -> ()
        n168 = local write "Source:"(w489) -> ()
        n169 = local write "Destination:"(w488) -> ()
        n170 = local write "page indicator"(w483) -> ()
      }
      frame "Stop" {
        n171 = control-ref of="This VI"() -> (w496:refnum<vi>)
        n172 = invoke class="VI" method="Default Vals.Reinit All"(reference=w496) -> (reference out=w495:refnum<vi>)  [unwired: 2 in, 2 out]
        n173 = Close Reference(reference=w495) -> ()  [unwired: 1 in, 1 out]
      }
      frame "Metadata to tree" {
        n174 = Unbundle By Name(w509) -> ("Active items.Recent ID"=w504:string, "Trees.Metadata"=w517:refnum<vi>)
        n175 = Not Equal?(x=w504, y="") -> (x != y?=w506:bool)
        n176 = Concatenate Strings("Metadata downloaded (id=" ("Communication.Project name"), w504, ")." ("string")) -> (w505:string)
        n177 = case shown="True" w506 {
          tunnel: w517 -> [w521 w531]
          tunnel: [w520 w530] -> w516
          tunnel: [w520 w529] -> w515
          tunnel: [w520 w528] -> w514
          tunnel: [w520 w527] -> w513
          tunnel: [w520 w526] -> w512
          tunnel: [w520 w525] -> _
          tunnel: w505 -> [_ w525]
          tunnel: w504 -> [_ w524]
          tunnel: w502 -> [w519 w523]
          tunnel: [w518 w522] -> w501
          frame False {
            w520 = ""
            n178 = invoke class="Tree (strict)" method="Edit Tree Items.Delete"(reference=w521, error in=w519) -> (error out=w518:errorcluster)  [unwired: 3 in, 4 out]
          }
          frame True {
            n179 = call "Rinocloud_HTTP_metadata_to_tree.vi"("error in (no error)"=w523, "JSON Tree Expanded Reference"=w531, "id"=w524) -> ("error out"=w522:errorcluster, "Notes"=w528:string, "Tags"=w529:string, "Name"=w530:string, "Status"=w532:T13)  [unwired: 3 in, 1 out]
            n180 = Unbundle By Name(w532) -> ("headers"=w527:string, "body"=w526:string)
          }
        }
        n181 = Bundle By Name(cluster=w509, "Update metadata.Name"=w516, "Update metadata.Tags"=w515, "Update metadata.Notes"=w514, "Communication.HTTP headers"=w513, "Communication.HTTP body"=w512) -> (w508:T3)
      }
      frame "Pagination" {
        n182 = Unbundle By Name(w538) -> ("Communication.HTTP ch body"=w546:string, "Pagination.limit"=w540:dbl, "Pagination.offset"=w539:dbl, "Pagination.next page refnum"=w534:refnum<vi>, "Pagination.previous page refnum"=w533:refnum<vi>)
        n183 = call "Rinocloud_pagination.vi"("error in (no error)"=w536, "HTTP body"=w546) -> ("error out"=w535:errorcluster, "pagination parameters"=w543:T12)  [unwired: 2 in]
        n184 = Unbundle By Name(w543) -> ("total"=w542:dbl)
        n185 = Bundle By Name(cluster=T12 {"limit"=15.0, "total"=0.0, "offset"=0.0, "count"=0.0} ("pagination parameters in"), "total"=w542, "limit"=w540, "offset"=w539) -> (w544:T12)
        n186 = call "Rinocloud_pagination_button_state.vi"("previous refnum"=w533, "next refnum"=w534, "pagination parameters in"=w544) -> ("pagination info"=w541:string)  [unwired: 8 in]
        n187 = Bundle By Name(cluster=w538, "Pagination.limit"=w540, "Pagination.offset"=w539, "Pagination.page indicator"=w541) -> (w537:T3)
      }
    }
    n188 = Or(x=w10, y="stop") -> (x .or. y?=w12:bool)
  }
  n189 = call <vilib>:"Simple Error Handler.vi"("error in (no error)"=w1) -> ()  [unwired: 4 in, 5 out]
